vi "Read ADC Current (SubVI).vi"(8 "error out":errorcluster, 9 "Param":dbl, 10 "Bool Refnum":refnum<vi>, 11 "VISAResourceName in":refnum<vi>) -> (0 "error out 2":errorcluster, 2 "Result":dbl)   [LabVIEW 2017]
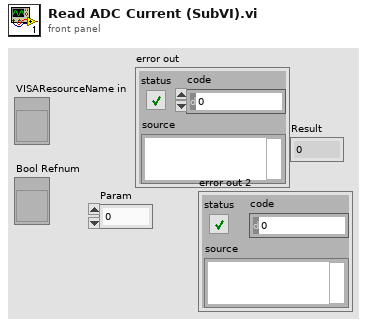
[diagram p1: front panel]
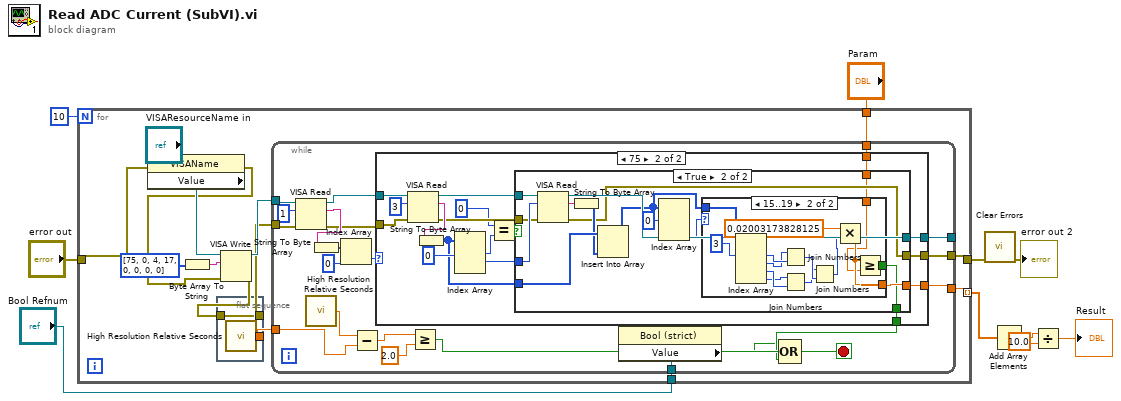
[diagram p0: block diagram]
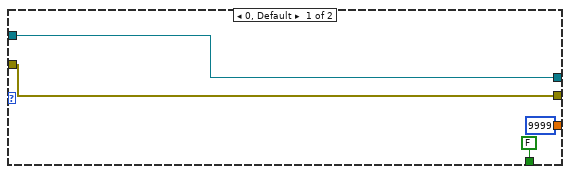
[diagram p2: hidden frame]
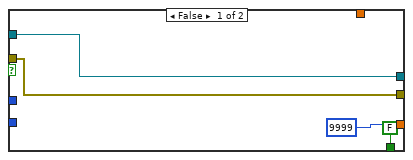
[diagram p3: hidden frame]
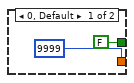
[diagram p4: hidden frame]
diagram:
  n1 = for {
    N: 10 -> [_]
    tunnel: [w14] -> w4 mode=indexing
    tunnel: "error out" -> [w24]
    tunnel: [w15] -> w8
    tunnel: "Param" -> [w13]
    tunnel: "Bool Refnum" -> [w11]
    n2 = property class="VISAName"(reference="VISAResourceName in", error in=w24) -> (error out=w16:errorcluster, "Value"=w17:refnum<visa-resource-name>)  [unwired: 1 out]
    n3 = Byte Array To String(unsigned byte array=u8[] [75, 0, 4, 17, 0, 0, 0, 0] ("appended array")) -> (string=w22:string)
    n4 = flat-sequence {
      tunnel: w23 -> [w102]
      tunnel: [w102] -> w20
      tunnel: [w101] -> w19
      frame #0 {
        n5 = call <vilib>:"High Resolution Relative Seconds.vi"() -> ("relative seconds"=w101:dbl)
      }
    }
    n6 = VISA Write(VISA resource name=w17, write buffer=w22, error in (no error)=w16) -> (VISA resource name out=w21:refnum<visa-resource-name>, error out=w23:errorcluster)  [unwired: 1 out]
    n7 = while {
      tunnel: w21 -> [w39]
      tunnel: w20 -> [w38]
      tunnel: [w37] -> _
      tunnel: [w36] -> w15
      tunnel: w19 -> [w34]
      tunnel: [w28] -> w14
      tunnel: w13 -> [w26]
      tunnel: w11 -> [w25]
      stop <- w30 stop-if-true
      n8 = VISA Read(VISA resource name=w39, byte count=u32 1, error in (no error)=w38) -> (VISA resource name out=w41:refnum<visa-resource-name>, read buffer=w42:string, error out=w40:errorcluster)  [unwired: 1 out]
      n9 = call <vilib>:"High Resolution Relative Seconds.vi"() -> ("relative seconds"=w35:dbl)
      n10 = String To Byte Array(string=w42) -> (unsigned byte array=w45:u8[])
      n11 = Index Array(array=w45, index=0) -> (element=w43:u8)
      n12 = Subtract(x=w35, y=w34) -> (x-y=w33:dbl)
      n13 = case shown="75" w43 {
        tunnel: [w50 w55] -> w36
        tunnel: w41 -> [w49 w64]
        tunnel: w40 -> [w50 w63]
        tunnel: [w49 w56] -> w37
        tunnel: [u32 9999 w53] -> w28
        tunnel: [FALSE w52] -> w29
        tunnel: w26 -> [_ w51]
        frame 0, Default {
        }
        frame 75 {
          n14 = VISA Read(VISA resource name=w64, byte count=u32 3, error in (no error)=w63) -> (VISA resource name out=w59:refnum<visa-resource-name>, read buffer=w67:string, error out=w58:errorcluster)  [unwired: 1 out]
          n15 = String To Byte Array(string=w67) -> (unsigned byte array=w57:u8[])
          n16 = Index Array(array=w57, index #1=0 ("index")) -> (element #1=w62:u8, element #2=w60:u8)  [unwired: 2 in, 1 out]
          n17 = Equal?(x=u8 0, y=w62) -> (x = y?=w61:bool)
          n18 = case shown="True" w61 {
            tunnel: [w70 w78] -> w55
            tunnel: w60 -> [_ w85]
            tunnel: w59 -> [w71 w84]
            tunnel: w58 -> [w70 w83]
            tunnel: w57 -> [_ w82]
            tunnel: [w71 w80] -> w56
            tunnel: [u32 9999 w74] -> w53
            tunnel: [FALSE w73] -> w52
            tunnel: w51 -> [_ w72]
            frame False {
            }
            frame True {
              n19 = VISA Read(VISA resource name=w84, byte count=w85, error in (no error)=w83) -> (VISA resource name out=w80:refnum<visa-resource-name>, read buffer=w79:string, error out=w78:errorcluster)  [unwired: 1 out]
              n20 = String To Byte Array(string=w79) -> (unsigned byte array=w81:u8[])
              n21 = Insert Into Array(array=w82, new element=w81) -> (w75:u8[])  [unwired: 1 in]
              n22 = Index Array(array=w75, index #1=0 ("index")) -> (element #3=w76:u8)  [unwired: 2 in, 2 out]
              n23 = case shown="15..19" w76 {
                tunnel: w75 -> [_ w99]
                tunnel: [u32 9999 w89] -> w74
                tunnel: [FALSE w90] -> w73
                tunnel: w72 -> [_ w88]
                frame 0, Default {
                }
                frame 15..19 {
                  n24 = Index Array(array=w99, index #1=3 ("index")) -> (element #1=w98:u8, element #2=w97:u8, element #3=w96:u8, element #4=w95:u8)  [unwired: 3 in]
                  n25 = Join Numbers(hi=w97, lo=w98) -> ((hi.lo)=w94:u16)
                  n26 = Join Numbers(hi=w95, lo=w96) -> ((hi.lo)=w93:u16)
                  n27 = Join Numbers(hi=w93, lo=w94) -> ((hi.lo)=w91:u32)
                  n28 = Multiply(x=0.02003173828125, y=w91) -> (x*y=w89:dbl)
                  n29 = Greater Or Equal?(x=w89, y=w88) -> (x >= y?=w90:bool)
                }
              }
            }
          }
        }
      }
      n30 = Greater Or Equal?(x=w33, y=2.0) -> (x >= y?=w31:bool)
      n31 = property on="Property Node" class="Bool (strict)"(reference=w25) -> ("Value"=w27:bool)  [unwired: 1 in, 2 out]
      n32 = Compound Arithmetic op=OR(w27, w31, w29) -> (w30:bool)
    }
  }
  n33 = call <vilib>:"Clear Errors.vi"("error in (no error)"=w8) -> ("error out"=→"error out 2":errorcluster)  [unwired: 5 in, 1 out]
  n34 = Add Array Elements(numeric array=w4) -> (sum=w6:dbl)
  n35 = Divide(x=w6, y=10.0) -> (x/y=→"Result":dbl)
